vi "dblvector_ave.vi"(11 "1DArray":dbl[](array[numeric])) -> (3 "Average":dbl)   [LabVIEW 2014]
doc: "Kiszámítja az 1DArray elemeinek átlagértékét. (Average)"
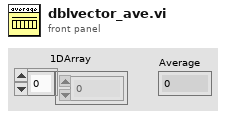
[diagram p1: front panel]
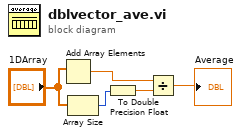
[diagram p0: block diagram]
diagram:
  n1 = Add Array Elements(numeric array="1DArray") -> (sum=w1:dbl)
  n2 = Array Size(array="1DArray") -> (size(s)=w3:i32)
  n3 = To Double Precision Float(number=w3) -> (double precision float=w4:dbl)
  n4 = Divide(x=w1, y=w4) -> (x/y=→"Average":dbl)
